vi "NUWARLoadCoordsTXT.vi"(0 "Input Path (dialog if empty)":path) -> (1 "Output Path (NotAPath if cancelled)":path, 2 "Buffer String":string)   [LabVIEW 2020]
doc: "Input Path is the file path of an ASCII file to read into Buffer String. If Input Path is empty (default value) or is Not A Path, the VI displays a File dialog box from which you can select a file. Output Path is the file path that was loaded and contained in Buffer String. Output Path is NotAPath if the user cancelled the operation.\n\nError 43 occurs if the user cancels the dialog."
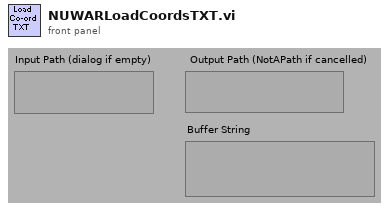
[diagram p1: front panel]
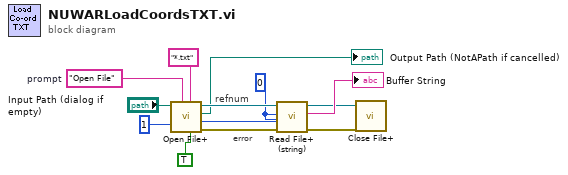
[diagram p0: block diagram]
diagram:
  w5 = i16 0 ("pos mode (rel. to begin)")
  w8 = "Open File"  # prompt
  # "error"
  # "refnum"
  n1 = call <vilib>:"Open File+.vi"("advisory dialog? (display:T)"=TRUE, "[pattern]"="*.txt", "prompt"=w8, "open mode (read-only:1)"=1, "file path (\" \")"="Input Path (dialog if empty)") -> ("error out"=w12:errorcluster, "file size (bytes)"=w4:i32, "file path"=→"Output Path (NotAPath if cancelled)":path, "refnum"=w7:refnum<file>)  [unwired: 3 in]
  n2 = call <vilib>:"Read File+ (string).vi"("count"=w4, "error in (no error)"=w12, "pos offset (bytes:0)"=w5, "pos mode (rel. to current:2)"=w5, "refnum"=w7) -> ("error out"=w10:errorcluster, "string"=→"Buffer String":string, "dup refnum"=w9:refnum<file>)  [unwired: 4 out]
  n3 = call <vilib>:"Close File+.vi"("error in (no error)"=w10, "refnum"=w9) -> ()  [unwired: 6 out]
